vi "Set BME G08.vi"(7 "DG Number":i32, 8 "error in (no error)":errorcluster, 11 "Settings":T1={"Channel A"={"Delay (µs)"=0.013000000000000001, "Pulse Width (µs)"=0.019, "Output Modulo"=300, "Output Offset"=0, "Go Signal"=16, "Polarity"=TRUE, "Terminate"=FALSE}, "Channel B"={"Delay (µs)"=0.032, "Pulse Width (µs)"=0.019, "Output Modulo"=300, "Output Offset"=0, "Go Signal"=16, "Polarity"=TRUE, "Terminate"=FALSE}, "Channel C"={"Delay (µs)"=0.0, "Pulse Width (µs)"=0.01, "Output Modulo"=300, "Output Offset"=0, "Go Signal"=16, "Polarity"=TRUE, "Terminate"=FALSE}, "Channel D"={"Delay (µs)"=0.01, "Pulse Width (µs)"=0.01, "Output Modulo"=300, "Output Offset"=0, "Go Signal"=16, "Polarity"=TRUE, "Terminate"=FALSE}, "Channel E"={"Delay (µs)"=0.039999999999999994, "Pulse Width (µs)"=0.01, "Output Modulo"=300, "Output Offset"=1, "Go Signal"=16, "Polarity"=TRUE, "Terminate"=FALSE, "Disconnect"=FALSE, "Onto MsBus"=FALSE, "Input Positive"=TRUE}, "Channel F"={"Delay (µs)"=0.04999999999999999, "Pulse Width (µs)"=0.01, "Output Modulo"=300, "Output Offset"=1, "Go Signal"=16, "Polarity"=TRUE, "Terminate"=FALSE, "Disconnect"=FALSE, "Onto MsBus"=FALSE, "Input Positive"=TRUE}, "Clock Enable"=TRUE, "Ocillator Divider"=2, "Trigger Divider"=1, "Trigger Multiplier"=4, "Clock Source"=3, "Trigger Terminate"=TRUE, "Gate Terminate"=TRUE, "Trigger Level"=0.2, "Gate Level"=0.0, "Gate Delay (µs)"=-1.0, "MS Bus"=1, "Internal Clock (µs)"=0.0083333, "Stop Trigger"=1, "Gate Divider"=0, "Force Trigger (µs)"=-1.0, "Step Back Time (µs)"=-1.0, "Burst Counter"=1, "Positive Gate"=TRUE, "Trigger Source"=TRUE, "Gate Type"=TRUE, "Synchronize Gate"=FALSE, "Trigger Slope"=TRUE, "Stop on Preset"=FALSE, "Reset When Done"=TRUE, "Trigger Enable"=TRUE, "Gate AB"=0, "Gate CD"=0, "Gate EF"=0} {"Gate EF" items=["Normal"=0, "EF_OR"=1048576, "EF_AND"=2097152, "EF_XOR"=3145728]; "Gate CD" items=["Normal"=0, "CD_OR"=262144, "CD_AND"=524288, "CD_XOR"=786432]; "Gate AB" items=["Normal"=0, "AB_OR"=65536, "AB_AND"=131072, "AB_XOR"=196608]; "Step Back Time (µs)" min=-1.0 format="%.6f"; "Force Trigger (µs)" min=-1.0 format="%.6f"; "Gate Delay (µs)" min=-1.0 format="%.6f"; "Internal Clock (µs)" min=0.0 format="%.6f"; "MS Bus" format="%04x" items=["Local Primary"=1, "Local Secondary"=2, "Local Force"=4, "Resynchronize"=8, "Master Primary"=16, "Master Secondary"=32, "Master Force"=64, "System Clock"=128, "Delay Clock"=256, "Inhibit Local"=512, "Start Local"=1024, "Start Bus"=2048, "Step Back Local"=4096, "Step Back Bus"=8192, "Enable From E"=65536, "Enable From F"=131072, "Enable From Bus"=262144]; "Gate Level" min=-2.5 max=2.5 format="%.3g"; "Trigger Level" min=-2.5 max=2.5 format="%.3f"; "Clock Source" items=["Internal Oscillator"=1, "External Trigger"=2, "Trigger & Oscillator"=3, "Master Slave Bus"=4]; "Trigger Multiplier" min=1; "Trigger Divider" min=1; "Ocillator Divider" min=1; "Channel F"."Go Signal" format="%04x" items=["Loc Prim"=1, "Loc Sec"=2, "Loc Force"=4, "Resynch"=8, "Mas Prim"=16, "Mas Sec"=32, "Mas Force"=64, "Sys Clock"=128, "Delay Clock"=256, "Inhibit Local"=512, "Start Local"=1024, "Start Bus"=2048, "Step Back Loc"=4096, "Step Back Bus"=8192, "From E"=65536, "From F"=131072, "From Bus"=262144]; "Channel F"."Pulse Width (µs)" min=0.0 max=8947840.0 format="%.6f"; "Channel F"."Delay (µs)" min=0.0 format="%.6f"; "Channel E"."Go Signal" format="%04x" items=["Loc Prim"=1, "Loc Sec"=2, "Loc Force"=4, "Resynch"=8, "Mas Prim"=16, "Mas Sec"=32, "Mas Force"=64, "Sys Clock"=128, "Delay Clock"=256, "Inhibit Local"=512, "Start Local"=1024, "Start Bus"=2048, "Step Back Loc"=4096, "Step Back Bus"=8192, "From E"=65536, "From F"=131072, "From Bus"=262144]; "Channel E"."Pulse Width (µs)" min=0.0 max=8947840.0 format="%.6f"; "Channel E"."Delay (µs)" min=0.0 format="%.6f"; "Channel D"."Go Signal" format="%04x" items=["Loc Prim"=1, "Loc Sec"=2, "Loc Force"=4, "Resynch"=8, "Mas Prim"=16, "Mas Sec"=32, "Mas Force"=64, "Sys Clock"=128, "Delay Clock"=256, "Inhibit Local"=512, "Start Local"=1024, "Start Bus"=2048, "Step Back Loc"=4096, "Step Back Bus"=8192, "From E"=65536, "From F"=131072, "From Bus"=262144]; "Channel D"."Pulse Width (µs)" min=0.0 max=8947840.0 format="%.6f"; "Channel D"."Delay (µs)" min=0.0 format="%.6f"; "Channel C"."Go Signal" format="%04x" items=["Loc Prim"=1, "Loc Sec"=2, "Loc Force"=4, "Resynch"=8, "Mas Prim"=16, "Mas Sec"=32, "Mas Force"=64, "Sys Clock"=128, "Delay Clock"=256, "Inhibit Local"=512, "Start Local"=1024, "Start Bus"=2048, "Step Back Loc"=4096, "Step Back Bus"=8192, "From E"=65536, "From F"=131072, "From Bus"=262144]; "Channel C"."Pulse Width (µs)" min=0.0 max=8947840.0 format="%.6f"; "Channel C"."Delay (µs)" min=0.0 format="%.6f"; "Channel B"."Go Signal" format="%04x" items=["Loc Prim"=1, "Loc Sec"=2, "Loc Force"=4, "Resynch"=8, "Mas Prim"=16, "Mas Sec"=32, "Mas Force"=64, "Sys Clock"=128, "Delay Clock"=256, "Inhibit Local"=512, "Start Local"=1024, "Start Bus"=2048, "Step Back Loc"=4096, "Step Back Bus"=8192, "From E"=65536, "From F"=131072, "From Bus"=262144]; "Channel B"."Pulse Width (µs)" min=0.0 max=8947840.0 format="%.6f"; "Channel B"."Delay (µs)" min=0.0 format="%.6f"; "Channel A"."Go Signal" format="%04x" items=["Loc Prim"=1, "Loc Sec"=2, "Loc Force"=4, "Resynch"=8, "Mas Prim"=16, "Mas Sec"=32, "Mas Force"=64, "Sys Clock"=128, "Delay Clock"=256, "Inhibit Local"=512, "Start Local"=1024, "Start Bus"=2048, "Step Back Loc"=4096, "Step Back Bus"=8192, "From E"=65536, "From F"=131072, "From Bus"=262144]; "Channel A"."Pulse Width (µs)" min=0.0 max=8947840.0 format="%.6f"; "Channel A"."Delay (µs)" min=0.0 format="%.6f"}) -> (0 "error out":errorcluster)   [LabVIEW 2009]
doc: "long Set_BME_G05(double FireFirst_T0, unsigned long OutputModulo_T0, BOOL Active_T0, BOOL Positive_T0, BOOL Terminate_T0, BOOL HighDrive_T0, double FireFirst_A, unsigned long OutputModulo_A, BOOL Active_A, BOOL Positive_A, BOOL Terminate_A, BOOL HighDrive_A, double FireFirst_B, unsigned long OutputModulo_B, BOOL Active_B, BOOL Positive_B, BOOL Terminate_B, BOOL HighDrive_B, BOOL Gate_AB, unsigned long OutputLevel, BOOL TriggerTerminate, BOOL ClockEnable, double InternalClock, double TriggerLevel, unsigned long PresetValue, unsigned long DivideBy, unsigned long ClockSource, unsigned long GateDivider, BOOL PositiveGate, BOOL InternalTrigger, BOOL InternalArm, BOOL SoftwareTrigger, BOOL RisingEdge, BOOL StopOnPreset, BOOL ResetWhenDone, BOOL TriggerEnable, long DG_Number);"
uses:
  Settings G08.ctl
  BME DLL/DelayGenerator.dll
panel:
  # "NOTICE -- YOU MUST LEAVE THIS NOTICE IN PLACE.  PER THE TERMS OF THE LICENSE BELOW, YOU MAY SUBLICENSE THIS SOFTWARE \nIN ANY WAY THAT DOES NOT CONFLICT WITH THIS LICENSE.\n\n### BSD License (http://www.opensource.org/licenses/bsd-license.php) Begin ###\n \nCopyright (c) 2011, Applied Energetics, http://www.appliedenergetics.com,\n                               Richard Schwerdtfeger, <rschwerdtfeger@appliedenergetics.com>\n\nAll rights reserved.\n\nRedistribution and use in source and binary forms, with or without modification, are permitted provided that the \nfollowing conditions are met:\n\n    * Redistributions of source code must retain the above copyright notice, this list of conditions and the following disclaimer.\n    * Redistributions in binary form must reproduce the above copyright notice, this list of conditions and the following disclaimer \n       in the documentation and/or other materials provided with the distribution.\n    * Neither the name of Richard Schwerdtfeger, Applied Energetics, Inc., nor the names of its contributors may be used to \n       endorse or promote products derived from this software without specific prior written permission.\n\nTHIS SOFTWARE IS PROVIDED BY THE COPYRIGHT HOLDERS AND CONTRIBUTORS \"AS IS\" AND ANY EXPRESS OR IMPLIED WARRANTIES, \nINCLUDING, BUT NOT LIMITED TO, THE IMPLIED WARRANTIES OF MERCHANTABILITY AND FITNESS FOR A PARTICULAR PURPOSE ARE \nDISCLAIMED. IN NO EVENT SHALL THE COPYRIGHT OWNER OR CONTRIBUTORS BE LIABLE FOR ANY DIRECT, INDIRECT, INCIDENTAL,\n SPECIAL, EXEMPLARY, OR CONSEQUENTIAL DAMAGES (INCLUDING, BUT NOT LIMITED TO, PROCUREMENT OF SUBSTITUTE GOODS OR \nSERVICES; LOSS OF USE, DATA, OR PROFITS; OR BUSINESS INTERRUPTION) HOWEVER CAUSED AND ON ANY THEORY OF LIABILITY, \nWHETHER IN CONTRACT, STRICT LIABILITY, OR TORT (INCLUDING NEGLIGENCE OR OTHERWISE) ARISING IN ANY WAY OUT OF THE USE \nOF THIS SOFTWARE, EVEN IF ADVISED OF THE POSSIBILITY OF SUCH DAMAGE.\n\n### BSD License End ###"
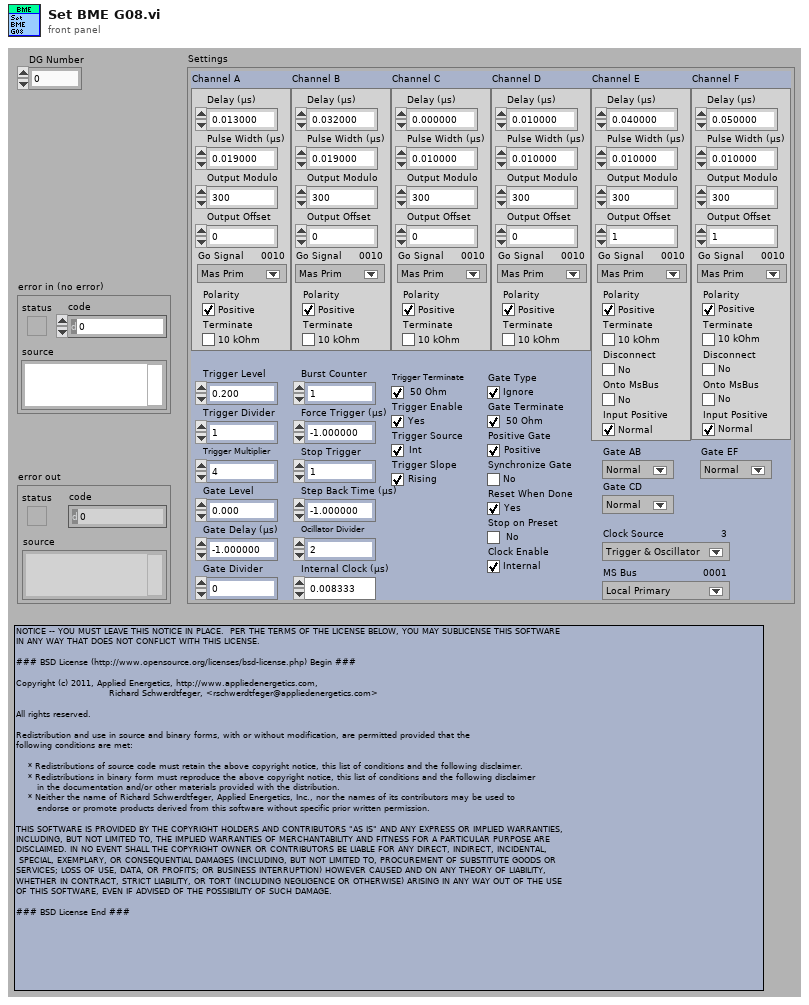
[diagram p1: front panel]
types:
  T1 = typedef "Settings G08.ctl" = cluster{"Channel A":cluster{"Delay (µs)":dbl, "Pulse Width (µs)":dbl, "Output Modulo":u32, "Output Offset":u32, "Go Signal":u32, "Polarity":bool, "Terminate":bool}, "Channel B":cluster{"Delay (µs)":dbl, "Pulse Width (µs)":dbl, "Output Modulo":u32, "Output Offset":u32, "Go Signal":u32, "Polarity":bool, "Terminate":bool}, "Channel C":cluster{"Delay (µs)":dbl, "Pulse Width (µs)":dbl, "Output Modulo":u32, "Output Offset":u32, "Go Signal":u32, "Polarity":bool, "Terminate":bool}, "Channel D":cluster{"Delay (µs)":dbl, "Pulse Width (µs)":dbl, "Output Modulo":u32, "Output Offset":u32, "Go Signal":u32, "Polarity":bool, "Terminate":bool}, "Channel E":cluster{"Delay (µs)":dbl, "Pulse Width (µs)":dbl, "Output Modulo":u32, "Output Offset":u32, "Go Signal":u32, "Polarity":bool, "Terminate":bool, "Disconnect":bool, "Onto MsBus":bool, "Input Positive":bool}, "Channel F":cluster{"Delay (µs)":dbl, "Pulse Width (µs)":dbl, "Output Modulo":u32, "Output Offset":u32, "Go Signal":u32, "Polarity":bool, "Terminate":bool, "Disconnect":bool, "Onto MsBus":bool, "Input Positive":bool}, "Clock Enable":bool, "Ocillator Divider":u32, "Trigger Divider":u32, "Trigger Multiplier":u32, "Clock Source":u32, "Trigger Terminate":bool, "Gate Terminate":bool, "Trigger Level":dbl, "Gate Level":dbl, "Gate Delay (µs)":dbl, "MS Bus":u32, "Internal Clock (µs)":dbl, "Stop Trigger":u32, "Gate Divider":u32, "Force Trigger (µs)":dbl, "Step Back Time (µs)":dbl, "Burst Counter":u32, "Positive Gate":bool, "Trigger Source":bool, "Gate Type":bool, "Synchronize Gate":bool, "Trigger Slope":bool, "Stop on Preset":bool, "Reset When Done":bool, "Trigger Enable":bool, "Gate AB":u32, "Gate CD":u32, "Gate EF":u32}
  T2 = cluster{"Delay (µs)":dbl, "Pulse Width (µs)":dbl, "Output Modulo":u32, "Output Offset":u32, "Go Signal":u32, "Polarity":bool, "Terminate":bool}
  T3 = cluster{"Delay (µs)":dbl, "Pulse Width (µs)":dbl, "Output Modulo":u32, "Output Offset":u32, "Go Signal":u32, "Polarity":bool, "Terminate":bool, "Disconnect":bool, "Onto MsBus":bool, "Input Positive":bool}
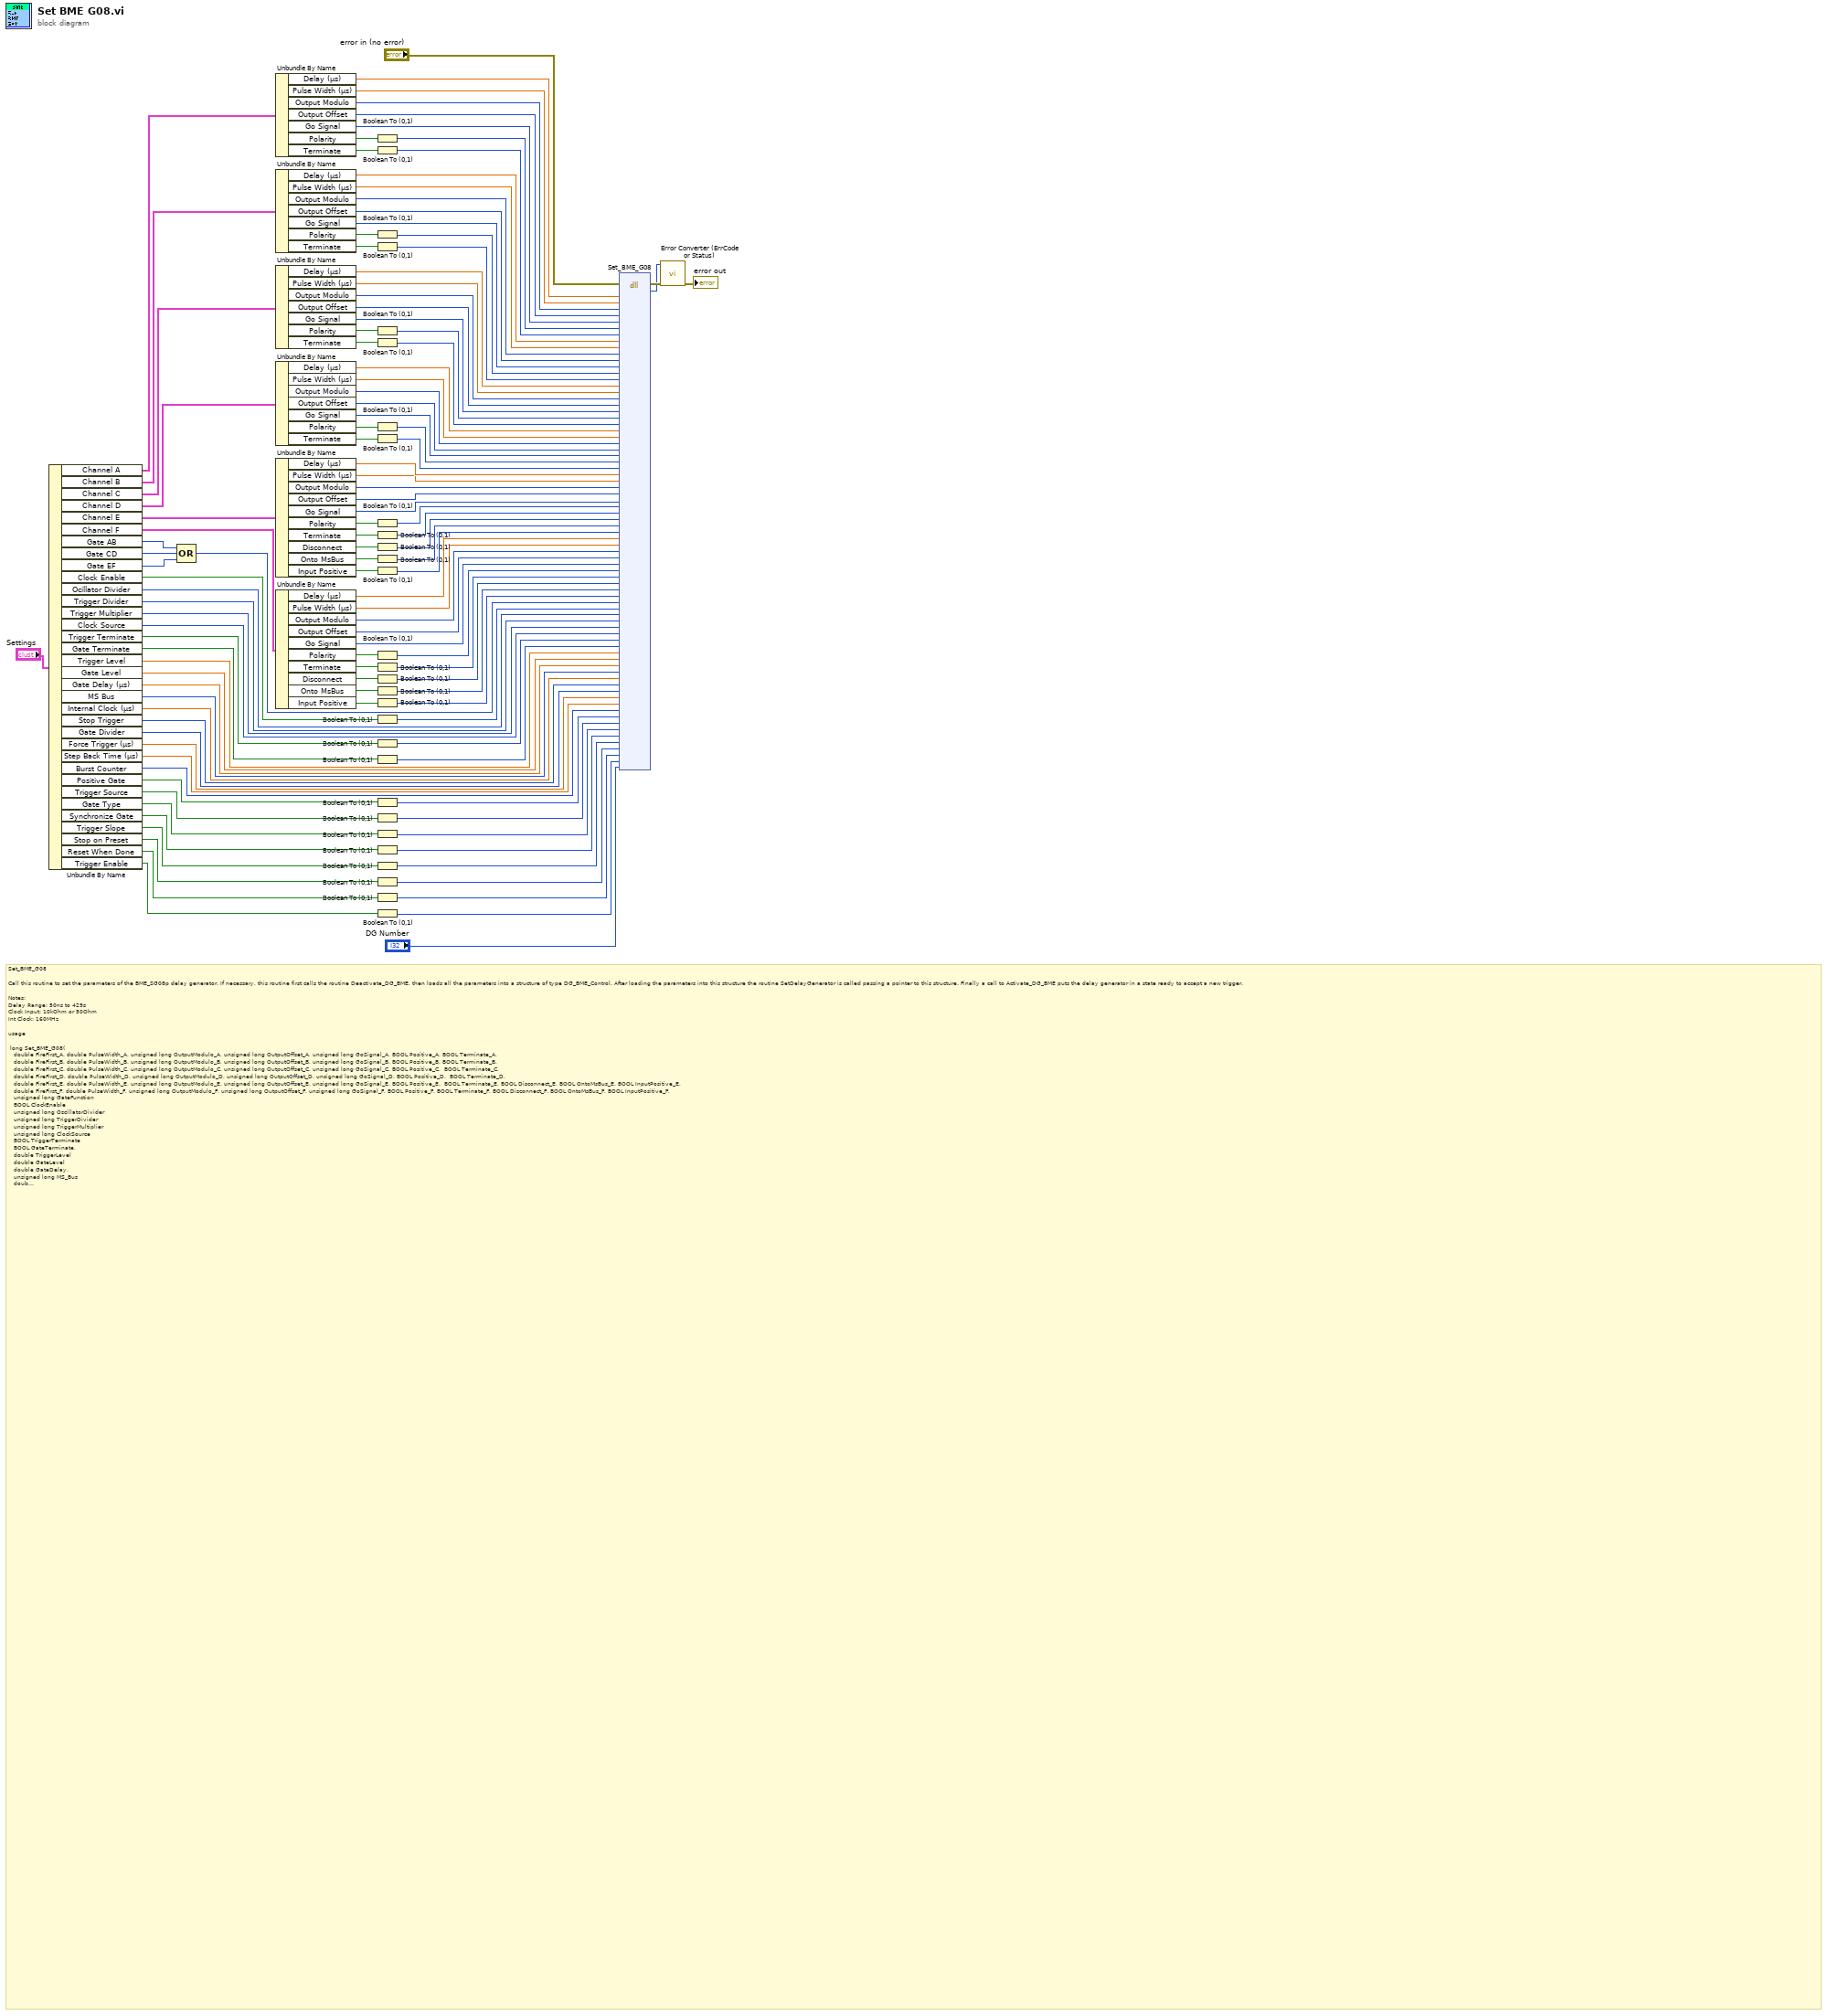
[diagram p0: block diagram]
diagram:
  # "Set_BME_G08\n\nCall this routine to set the parameters of the BME_SG08p delay generator. If necessary, this routine first calls the routine Deactivate_DG_BME, then loads all the parameters into a structure of type DG_BME_Control. After loading the parameters into this structure the routine SetDelayGenerator is called passing a pointer to this structure. Finally a call to Activate_DG_BME puts the delay generator in a state ready to accept a new trigger.\n\nNotes: \nDelay Range: 50ns to 429s\nClock Input: 10kOhm or 50Ohm\nInt Clock: 160MHz\n\nusage\n\n long Set_BME_G08(\n   double FireFirst_A, double PulseWidth_A, unsigned long OutputModulo_A, unsigned long OutputOffset_A, unsigned long GoSignal_A, BOOL Positive_A, BOOL Terminate_A, \n   double FireFirst_B, double PulseWidth_B, unsigned long OutputModulo_B, unsigned long OutputOffset_B, unsigned long GoSignal_B, BOOL Positive_B, BOOL Terminate_B,\n   double FireFirst_C, double PulseWidth_C, unsigned long OutputModulo_C, unsigned long OutputOffset_C, unsigned long GoSignal_C, BOOL Positive_C,  BOOL Terminate_C,\n   double FireFirst_D, double PulseWidth_D, unsigned long OutputModulo_D, unsigned long OutputOffset_D, unsigned long GoSignal_D, BOOL Positive_D,  BOOL Terminate_D,\n   double FireFirst_E, double PulseWidth_E, unsigned long OutputModulo_E, unsigned long OutputOffset_E, unsigned long GoSignal_E, BOOL Positive_E,  BOOL Terminate_E, BOOL Disconnect_E, BOOL OntoMsBus_E, BOOL InputPositive_E,\n   double FireFirst_F, double PulseWidth_F, unsigned long OutputModulo_F, unsigned long OutputOffset_F, unsigned long GoSignal_F, BOOL Positive_F, BOOL Terminate_F, BOOL Disconnect_F, BOOL OntoMsBus_F, BOOL InputPositive_F,\n   unsigned long GateFunction\n   BOOL ClockEnable\n   unsigned long OscillatorDivider\n   unsigned long TriggerDivider\n   unsigned long TriggerMultiplier\n   unsigned long ClockSource\n   BOOL TriggerTerminate\n   BOOL GateTerminate,\n   double TriggerLevel\n   double GateLevel\n   double GateDelay,\n   unsigned long MS_Bus\n   double InternalClock\n   unsigned long PresetValue,\n   unsigned long GateDivider\n   double ForceTrigger\n   double StepBackTime,\n   unsigned long BurstCounter\n   BOOL PositiveGate\n   BOOL InternalTrigger,\n   BOOL IgnoreGate\n   BOOL SynchronizeGate\n   BOOL RisingEdge,\n   BOOL StopOnPreset\n   BOOL ResetWhenDone,\n   BOOL TriggerEnable\n   long DG_Number);\n\n\nparameters\n\n\tChannel\n\t   FireFirst:\t\ttime after the main trigger in µsec, when the specified output should be set\n\t   PulseWidth:\t\tlength of the output pulse in µsec\n\t  \tOutputModulo:\t\tfor every number of trigger events specified in this variable, only one pulse will actually be output at the connector of the delay generator.\n\t  \tOutputOffset:\t\tthis vairable specifies the offset when starting to count the trigger events until a pulse comes from the output connector.\n\t  \tGoSignal:\t\tthe bits of this unsigned long parameter define which of the trigger signals available starts this channel. These signals can or’ed. The corresponding constants are defined in ‘’DG_Data.h’’.)\n\t  \tPositive:\t\tTRUE to specify a positive output polarity, otherwise FALSE\n\t  \tTerminate:\t\tTRUE to specify an internal 50 ohm termination on the specified output,otherwise FALSE\n        Chan E & F\n\t  \t    Disconnect:\t\tset this flag to TRUE for channels E or F of the BME_SG08 card if the  output driver should be disconnected from the connector at the slot. The output driver must be disconnected, if some external signal is to be entered.\n\t    \t  OntoMsBus:\t\tset this flag to TRUE for channels E or F of the BME_SG08 card if the \tsignal from this connector should be placed onto the master/slave bus for use at the slave cards\n\t    \t  InputPositive:\t\tset this flag to FALSE for channels E or F of the BME_SG08 card if the signal should be inverted before it is used e.g. as enable.\n\n\t  \t--------------------------------------------------------------\n\n\t  \tGateFunction: this parameter defines how the six outputs A,B...F are combined in pairs AB, CD and EGF to form a gated output or wheteher they should fire independently. (The values of the parameter GateFunction are defined in ‘’DG_Data.h’’.)\n\t  \tClockEnable: this flag must be set to enable the clock circuit\n\t  \tOscillatorDivider: the oscillator signal is divided by this value. Actually, the external oscillator is first multiplied by 2 before it is divided by this value.\n\t  \tTriggerDivider: the signal coming from the trigger input connector is divided by this value. \n\t  \tTriggerMultiplier: the signal coming from the trigger input connector is multiplied by this value. When the frequency of the signal entered at the trigger input connector is less than 10MHz, this input signal must be transformed to a higher frequency. Powers of 2 are allowed up to 128.\n\t  \tClockSource: the source of the clock signal, can be the crystal oscillator or a signal fedto the external trigger input. (The constants for this variable, CrystalOscillator or TriggerInput, are defined in ‘’DG_Data.h’’.)\n\t  \tTriggerTerminate: TRUE to specify an internal 50 ohm termination on the trigger input, otherwise FALSE\n\t  \tGateTerminate: TRUE to specify an internal 50 ohm termination on the gate input, otherwise FALSE\n\t  \tTriggerLevel: Voltage of the trigger threshold. Can be varied from -2.5V to +2.5V\n\t  \tGateLevel: Voltage of the gate threshold. Can be varied from -2.5V to +2.5V\n\t  \tGateDelay: when an external gate is detected, the force counter is immediately set to the beginning of its count. Since it is possible that the force trigger has just fired and corresponding delays are still active, wait this time until a trigger event by the gate circuit is generated. \n\t  \tMS_Bus: only one bit of this unsigned long parameter is used: (The corresponding constants are defined in ‘’DG_Data.h’’.)\n\t  \tInternalClock: period of the internal clock in µsec.\n\t  \tPresetValue: this will disable the trigger circuit after this number of trigger signals has occurred, provided the StopOnPreset flag is set.\n\t  \tGateDivider: the external gate signal will be divided by this number.\n\t  \tForceTrigger: time in µsec after a valid trigger event, that the delay generator will be triggered again internally.\n\t  \tStepBackTime: time in µsec after a valid trigger event, that the delay lists will be stepped back according to the value pointed to by the step back array.\n\t  \tBurstCounter: entering a nonzero number into this control will generate a corresponding number of triggers after a valid external trigger event. The time difference between trigger events of this burst is defined by the inhibit time.\n\t  \tPositiveGate: set this flag to TRUE, if a positive signal on the external gate input should enable the trigger circuit, otherwise FALSE. Note that the TriggerEnable flag is or’ed with the external gate signal. Only when the TriggerEnable flag is set FALSE, the trigger circuit can be enabled by the external gate signal.\n\t  \tInternalTrigger: if this flag is set the BME_G02 will be triggered by its internal clock, (provided it is jumpered as a master module).\n\t  \tIgnoreGate: set this flag to TRUE, if gate signals should be ignored during the time the InhibitTrigger counter has not elapsed yet. If this flag is set to FALSE, all valid gate signals from the time the outputs of the delay generator have been reset will be memorized, causing a trigger after the InhibitTrigger counter elapses.\n\t  \tSynchronize Gate: set this flag to TRUE, if the width of the gate signal should be measured and this measured width used for determining the time difference between primary and secondary trigger events. Note that the primary trigger is the trigger event which is directly specified by the setting of the trigger controls. If the rising edge of the gate signal causes the primary trigger event, then the secondary trigger event is caused by the falling edge of the trigger signal.\n\t  \tRisingEdge: if none of the flags InternalTrigger or SoftwareTrigger are set and this module is jumpered as master, the BME_G02 will be triggered by the rising edge of a signal applied to its external connector.\n\t  \tStopOnPreset: if this flag is set, the BME_G02 will disable its trigger circuit when the number of triggers prescribed by PresetValue has been reached. Modules slaved to a master will also stop at this point.\n\t  \tResetWhenDone: if this flag is set, all outputs from master and slave(s) will be reset to their untriggered states 2 µsec after the last delay of master and slave(s) has elapsed. This function is controlled by the master module. If this flag is not set, all modules, master and slave(s) have to be individually reset by calling the two routines Deactivate_DG_BME and Activate_DG_BME (in that order).\n\t  \tTriggerEnable: this flag must be set to enable the trigger circuit. This signal is or'ed withthe signal coming from the external gate input. Actually, the rising edge of the (divided) gate signal clocks a flip-flop allowing a trigger. After a trigger has occurred, the flip-flop is reset.\n\t  \tDG_Number:\t\tThe number of the delay generator as assigned by the Initialize_DG_BME routine\n\nreturn value\n\n0:  success\n2:  DG_Number is out of range\n3:  the FireFirst time of an output is negative while the Active flag is TRUE.\n4:  more than one of the flags InternalTrigger, InternalArm, and SoftwareTrigger have both been set\n5:  one or more delay time(s) is specified too long\n6:  parameter ‘OutputLevel’ has been passed with illegal value. (See DG_Data.h)\n7:  parameter ‘ClockSource’ has been passed with illegal value. (See DG_Data.h)"
  n1 = Unbundle By Name("Settings") -> ("Channel A"=w106:T2, "Channel B"=w93:T2, "Channel C"=w92:T2, "Channel D"=w91:T2, "Channel E"=w90:T3, "Channel F"=w89:T3, "Gate AB"=w4:u32, "Gate CD"=w3:u32, "Gate EF"=w2:u32, "Clock Enable"=w107:bool, "Ocillator Divider"=w43:u32, "Trigger Divider"=w42:u32, "Trigger Multiplier"=w41:u32, "Clock Source"=w40:u32, "Trigger Terminate"=w108:bool, "Gate Terminate"=w109:bool, "Trigger Level"=w37:dbl, "Gate Level"=w36:dbl, "Gate Delay (µs)"=w35:dbl, "MS Bus"=w34:u32, "Internal Clock (µs)"=w33:dbl, "Stop Trigger"=w32:u32, "Gate Divider"=w31:u32, "Force Trigger (µs)"=w30:dbl, "Step Back Time (µs)"=w29:dbl, "Burst Counter"=w28:u32, "Positive Gate"=w110:bool, "Trigger Source"=w111:bool, "Gate Type"=w112:bool, "Synchronize Gate"=w113:bool, "Trigger Slope"=w114:bool, "Stop on Preset"=w115:bool, "Reset When Done"=w116:bool, "Trigger Enable"=w117:bool)
  n2 = Compound Arithmetic op=OR(w4, w3, w2) -> (w1:u32)
  n3 = Unbundle By Name(w106) -> ("Delay (µs)"=w86:dbl, "Pulse Width (µs)"=w85:dbl, "Output Modulo"=w84:u32, "Output Offset"=w83:u32, "Go Signal"=w82:u32, "Polarity"=w105:bool, "Terminate"=w104:bool)
  n4 = Unbundle By Name(w93) -> ("Delay (µs)"=w79:dbl, "Pulse Width (µs)"=w78:dbl, "Output Modulo"=w77:u32, "Output Offset"=w76:u32, "Go Signal"=w75:u32, "Polarity"=w102:bool, "Terminate"=w103:bool)
  n5 = Unbundle By Name(w92) -> ("Delay (µs)"=w72:dbl, "Pulse Width (µs)"=w71:dbl, "Output Modulo"=w70:u32, "Output Offset"=w69:u32, "Go Signal"=w68:u32, "Polarity"=w98:bool, "Terminate"=w99:bool)
  n6 = Unbundle By Name(w91) -> ("Delay (µs)"=w65:dbl, "Pulse Width (µs)"=w64:dbl, "Output Modulo"=w63:u32, "Output Offset"=w62:u32, "Go Signal"=w61:u32, "Polarity"=w101:bool, "Terminate"=w100:bool)
  n7 = Unbundle By Name(w90) -> ("Delay (µs)"=w58:dbl, "Pulse Width (µs)"=w57:dbl, "Output Modulo"=w56:u32, "Output Offset"=w55:u32, "Go Signal"=w54:u32, "Polarity"=w97:bool, "Terminate"=w96:bool, "Disconnect"=w19:bool, "Onto MsBus"=w18:bool, "Input Positive"=w17:bool)
  n8 = Unbundle By Name(w89) -> ("Delay (µs)"=w51:dbl, "Pulse Width (µs)"=w50:dbl, "Output Modulo"=w49:u32, "Output Offset"=w48:u32, "Go Signal"=w47:u32, "Polarity"=w94:bool, "Terminate"=w95:bool, "Disconnect"=w13:bool, "Onto MsBus"=w12:bool, "Input Positive"=w11:bool)
  n9 = Boolean To (0,1)(Boolean=w105) -> (0, 1=w81:i16)
  n10 = Boolean To (0,1)(Boolean=w104) -> (0, 1=w80:i16)
  n11 = Boolean To (0,1)(Boolean=w102) -> (0, 1=w74:i16)
  n12 = Boolean To (0,1)(Boolean=w103) -> (0, 1=w73:i16)
  n13 = Boolean To (0,1)(Boolean=w98) -> (0, 1=w67:i16)
  n14 = Boolean To (0,1)(Boolean=w99) -> (0, 1=w66:i16)
  n15 = Boolean To (0,1)(Boolean=w101) -> (0, 1=w60:i16)
  n16 = Boolean To (0,1)(Boolean=w100) -> (0, 1=w59:i16)
  n17 = Boolean To (0,1)(Boolean=w97) -> (0, 1=w53:i16)
  n18 = Boolean To (0,1)(Boolean=w96) -> (0, 1=w52:i16)
  n19 = Boolean To (0,1)(Boolean=w19) -> (0, 1=w14:i16)
  n20 = Boolean To (0,1)(Boolean=w18) -> (0, 1=w15:i16)
  n21 = Boolean To (0,1)(Boolean=w17) -> (0, 1=w16:i16)
  n22 = Boolean To (0,1)(Boolean=w94) -> (0, 1=w46:i16)
  n23 = Boolean To (0,1)(Boolean=w95) -> (0, 1=w45:i16)
  n24 = Boolean To (0,1)(Boolean=w13) -> (0, 1=w8:i16)
  n25 = Boolean To (0,1)(Boolean=w12) -> (0, 1=w9:i16)
  n26 = Boolean To (0,1)(Boolean=w11) -> (0, 1=w10:i16)
  n27 = Boolean To (0,1)(Boolean=w107) -> (0, 1=w44:i16)
  n28 = Boolean To (0,1)(Boolean=w108) -> (0, 1=w39:i16)
  n29 = Boolean To (0,1)(Boolean=w109) -> (0, 1=w38:i16)
  n30 = Boolean To (0,1)(Boolean=w110) -> (0, 1=w27:i16)
  n31 = Boolean To (0,1)(Boolean=w111) -> (0, 1=w26:i16)
  n32 = Boolean To (0,1)(Boolean=w112) -> (0, 1=w25:i16)
  n33 = Boolean To (0,1)(Boolean=w113) -> (0, 1=w24:i16)
  n34 = Boolean To (0,1)(Boolean=w114) -> (0, 1=w23:i16)
  n35 = Boolean To (0,1)(Boolean=w115) -> (0, 1=w22:i16)
  n36 = Boolean To (0,1)(Boolean=w116) -> (0, 1=w21:i16)
  n37 = Boolean To (0,1)(Boolean=w117) -> (0, 1=w20:i16)
  n38 = dll-call lib="C:/Dokumente und Einstellungen/A2.5/Desktop/POLARIS BME DG/BME DLL/DelayGenerator.dll" fn="Set_BME_G08"(error in="error in (no error)", "FireFirst_A"=w86, "PulseWidth_A"=w85, "OutputModulo_A"=w84, "OutputOffset_A"=w83, "GoSignal_A"=w82, "Positive_A"=w81, "Terminate_A"=w80, "FireFirst_B"=w79, "PulseWidth_B"=w78, "OutputModulo_B"=w77, "OutputOffset_B"=w76, "GoSignal_B"=w75, "Positive_B"=w74, "Terminate_B"=w73, "FireFirst_C"=w72, "PulseWidth_C"=w71, "OutputModulo_C"=w70, "OutputOffset_C"=w69, "GoSignal_C"=w68, "Positive_C"=w67, "Terminate_C"=w66, "FireFirst_D"=w65, "PulseWidth_D"=w64, "OutputModulo_D"=w63, "OutputOffset_D"=w62, "GoSignal_D"=w61, "Positive_D"=w60, "Terminate_D"=w59, "FireFirst_E"=w58, "PulseWidth_E"=w57, "OutputModulo_E"=w56, "OutputOffset_E"=w55, "GoSignal_E"=w54, "Positive_E"=w53, "Terminate_E"=w52, "Disconnect_E"=w14, "OntoMsBus_E"=w15, "InputPositive_E"=w16, "FireFirst_F"=w51, "PulseWidth_F"=w50, "OutputModulo_F"=w49, "OutputOffset_F"=w48, "GoSignal_F"=w47, "Positive_F"=w46, "Terminate_F"=w45, "Disconnect_F"=w8, "OntoMsBus_F"=w9, "InputPositive_F"=w10, "GateFunction"=w1, "ClockEnable"=w44, "OscillatorDivider"=w43, "TriggerDivider"=w42, "TriggerMultiplier"=w41, "ClockSource"=w40, "TriggerTerminate"=w39, "GateTerminate"=w38, "TriggerLevel"=w37, "GateLevel"=w36, "GateDelay"=w35, "MS_Bus"=w34, "InternalClock"=w33, "PresetValue"=w32, "GateDivider"=w31, "ForceTrigger"=w30, "StepBackTime"=w29, "BurstCounter"=w28, "PositiveGate"=w27, "InternalTrigger"=w26, "IgnoreGate"=w25, "SynchronizeGate"=w24, "RisingEdge"=w23, "StopOnPreset"=w22, "ResetWhenDone"=w21, "TriggerEnable"=w20, "DG_Number"="DG Number") -> (error out=w88:errorcluster, "return type"=w87:i32)  [unwired: 77 in, 1 out]
  n39 = call "Error Converter (ErrCode or Status).vi"("error in (no error)"=w88, "error code"=w87) -> ("error out"=→"error out":errorcluster)  [unwired: 9 out]
